vi "Check_file_header.vi"(0 "Filename":path, 7 "Present Channels only":bool, 9 "Present Channels":string[](array[string]), 11 "Start of read offset (chars.: 0)":i32) -> (3 "File Channels":string[](array[string]), 4 "exists?":bool, 6 "Merged Channels":string[](array[string]), 8 "Start of data (bytes)":i32, 10 "No of bytes/row (approx)":i32, 14 "Current file size (bytes)":i32, 15 "Merged?":bool)   [LabVIEW 2010]
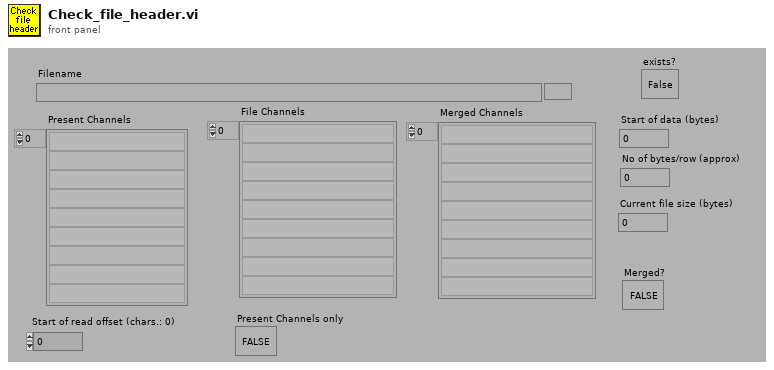
[diagram p1: front panel]
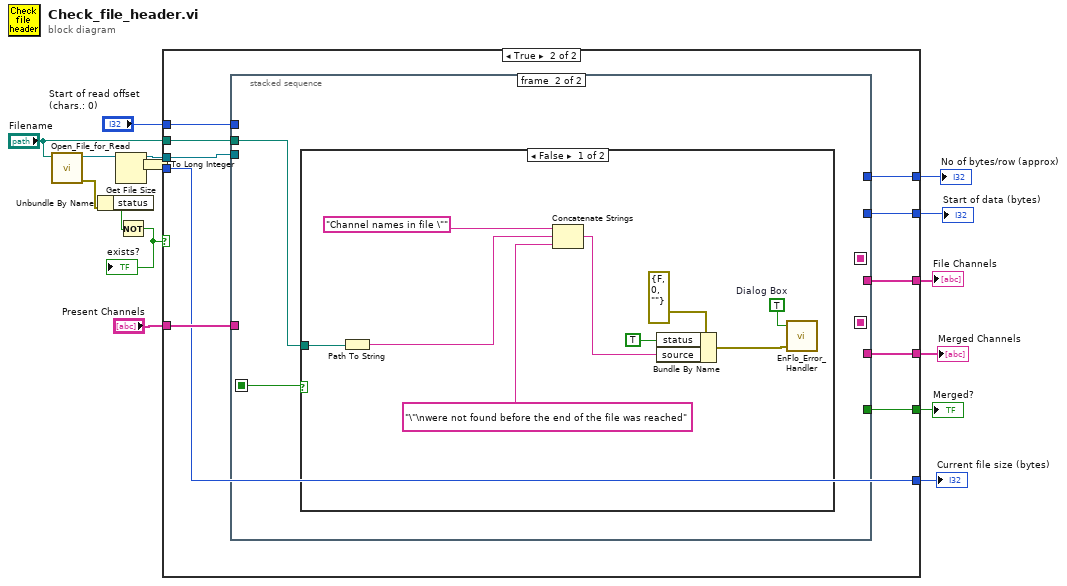
[diagram p0: block diagram]
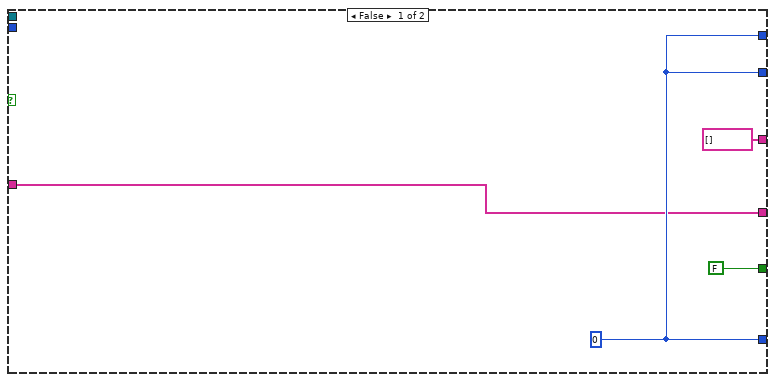
[diagram p2: hidden frame]
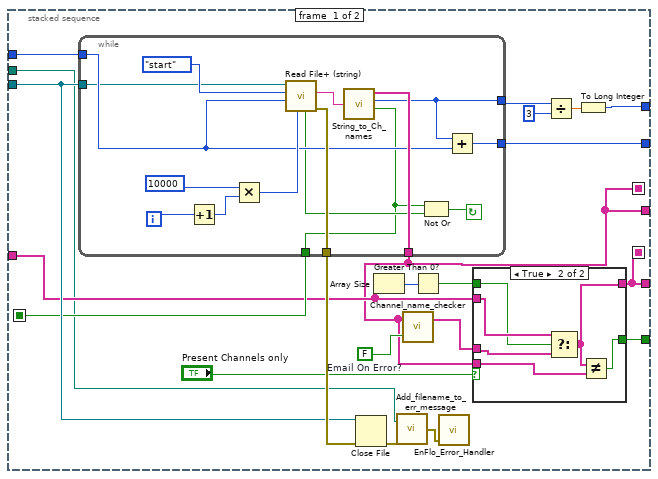
[diagram p3: hidden frame]
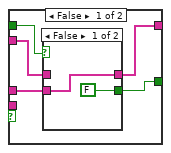
[diagram p4: hidden frame]
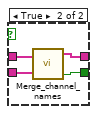
[diagram p5: hidden frame]
diagram:
  n1 = call "Open_File_for_Read.vi"("file path"="Filename") -> ("error out"=w10:errorcluster, "refnum"=w2:refnum<file>)  [unwired: 1 in, 8 out]
  n2 = Unbundle By Name(w10) -> ("status"=w13:bool)
  n3 = Get File Size(file=w2) -> (refnum out=w9:refnum<file>, size (in bytes)=w1:i64)  [unwired: 1 in, 1 out]
  n4 = Not(x=w13) -> (.not. x?=w12:bool)
  "exists?" <- w12
  n5 = To Long Integer(number=w1) -> (32bit integer=w8:i32)
  n6 = case shown="True" w12 {
    tunnel: [w17 w29] -> w16
    tunnel: "Present Channels" -> [w17 w30]
    tunnel: [FALSE ("Merged?") w28] -> w14
    tunnel: "Filename" -> [_ w22]
    tunnel: w9 -> [_ w23]
    tunnel: w8 -> [_ w24]
    tunnel: "Start of read offset (chars.: 0)" -> [_ w27]
    tunnel: [w19 w26] -> w6
    tunnel: [w19 w25] -> w5
    tunnel: [w19 w24] -> w4
    tunnel: [string[] [] ("Ch names") w21] -> w3
    frame False {
      w19 = 0 ("offset")
    }
    frame True {
      n7 = stacked-sequence {
        seq-local: [w43 _] -> [_ w85]
        seq-local: [w34 _] -> [_ _]
        seq-local: [w36 _] -> [_ _]
        tunnel: w30 -> [w39 _]
        tunnel: [w36 _] -> w29
        tunnel: [w35 _] -> w28
        tunnel: w27 -> [w51 _]
        tunnel: [w47 _] -> w26
        tunnel: [w46 _] -> w25
        tunnel: w23 -> [w44 _]
        tunnel: w22 -> [w31 w84]
        tunnel: [w34 _] -> w21
        frame #0 {
          w41 = FALSE  # Email On Error?
          n8 = while {
            tunnel: [w52] -> w43
            tunnel: [w57] -> w50
            tunnel: w51 -> [w58]
            tunnel: [w60] -> w45
            tunnel: [w61] -> w46
            tunnel: [w62] -> w34
            tunnel: w44 -> [w56]
            i -> [w54]
            stop <- w55 continue-if-true
            n9 = Increment(x=w54) -> (x+1=w59:i32)
            n10 = Multiply(x=10000 ("count"), y=w59) -> (x*y=w64:i32)
            n11 = call <vilib>:"Read File+ (string).vi"("count"=w64, "pos offset (bytes:0)"=w58, "pos mode (rel. to current:2)"=enum16{"start", "end", "current"}."start" ("pos mode (0:2)"), "refnum"=w56) -> ("error out"=w60:errorcluster, "string"=w63:string, "EOF?"=w53:bool)  [unwired: 1 in, 4 out]
            n12 = call "String_to_Ch_names.vi"("Spreadsheet string"=w63) -> ("Ch names"=w62:string[], "Title length (Bytes)"=w57:i32, "Title Rows Found?"=w52:bool)  [unwired: 1 out]
            n13 = Not Or(1:w53, 2:w52) -> (0:w55:bool)
            n14 = Add(x=w57, y=w58) -> (x+y=w61:i32)
          }
          n15 = Close File(refnum=w44, error in=w45) -> (error out=w33:errorcluster)  [unwired: 1 out]
          n16 = Array Size(array=w39) -> (size(s)=w40:i32)
          n17 = call "Add_filename_to_err_message.vi"("error in (no error)"=w33, "Path"=w31) -> ("error out"=w32:errorcluster)
          n18 = call "Channel_name_checker.vi"("Email On Error?"=w41, "Channel names"=w34) -> ("Channel names Out"=w37:string[])  [unwired: 1 out]
          n19 = Greater Than 0?(x=w40) -> (x > 0?=w38:bool)
          n20 = call "EnFlo_Error_Handler.vi"("error in (no error)"=w32) -> ()  [unwired: 2 in, 3 out]
          n21 = case shown="True" "Present Channels only" {
            tunnel: w39 -> [w71 w83]
            tunnel: [w70 w80] -> w36
            tunnel: w37 -> [w69 w81]
            tunnel: w38 -> [w68 w82]
            tunnel: [w67 w78] -> w35
            tunnel: w34 -> [_ w79]
            frame False {
              n22 = case shown="False" w68 {
                tunnel: w71 -> [_ w77]
                tunnel: [w73 w76] -> w70
                tunnel: [FALSE ("Merged?") w75] -> w67
                tunnel: w69 -> [w73 w74]
                frame False {
                }
                frame True {
                  n23 = call "Merge_channel_names.vi"("Preferred Channel array"=w77, "Channel array"=w74) -> ("Merged Channels"=w76:string[], "Channel Array Changed?"=w75:bool)  [unwired: 1 out]
                }
              }
            }
            frame True {
              n24 = Select(t=w83, s=w82, f=w81) -> (s? t:f=w80:string[])
              n25 = Not Equal?(x=w80, y=w79) -> (x != y?=w78:bool)
            }
          }
          n26 = Divide(x=w50, y=3) -> (x/y=w48:dbl)
          n27 = To Long Integer(number=w48) -> (32bit integer=w47:i32)
        }
        frame #1 {
          n28 = case shown="False" w85 {
            tunnel: w84 -> [w92 _]
            frame False {
              w89 = TRUE  # Dialog Box
              n29 = Path To String(path=w92) -> (string=w91:string)
              n30 = Concatenate Strings("Channel names in file \"" ("message"), w91, "\"\nwere not found before the end of the file was reached" ("message")) -> (w87:string)
              n31 = Bundle By Name(cluster=errorcluster {"status"=FALSE, "code"=0, "source"=""} ("error in (no error)"), "status"=TRUE ("Bundle Element"), "source"=w87) -> (w86:errorcluster)
              n32 = call "EnFlo_Error_Handler.vi"("error in (no error)"=w86, "Dialog Box (T)"=w89) -> ()  [unwired: 1 in, 3 out]
            }
            frame True {
            }
          }
        }
      }
    }
  }
  "Merged?" <- w14
  "Merged Channels" <- w16
  "Current file size (bytes)" <- w4
  "Start of data (bytes)" <- w5
  "No of bytes/row (approx)" <- w6
  "File Channels" <- w3
